vi "CALC_Fwd_adjust_TTL_pulse_length_according_to_stim_type_2.vi"(9 "Condition":refnum<class "Reward_Condition.lvclass">, 10 "Calibration parameters":T1 {"True frame time, s" format="%.10g"; "Disp. calibration info"."Speed, µl per ms" format="%.3g"; "True FPS" format="%.10g"; "Timing calibration sw/hw" format="%.10g"}, 11 "TTL pulse length ref in":refnum<vi>) -> ()   [LabVIEW 2018, in "Tracker.lvlib"]
uses:
  Tracker.lvlib
  Controls/CTL_Calibration_parameters.ctl
  Controls/CTL_Dispenser_calibration_info.ctl
  Classes/Reward_Condition/Reward_Condition.lvclass
  Classes/Reward_Condition/Reward_Condition.lvclass/Reward_Condition.ctl
  Classes/Reward_Condition/Read Response destination.vi
  Classes/Reward_Condition/Read Response length, ms.vi
  Classes/Reward_Condition/Read Response type.vi
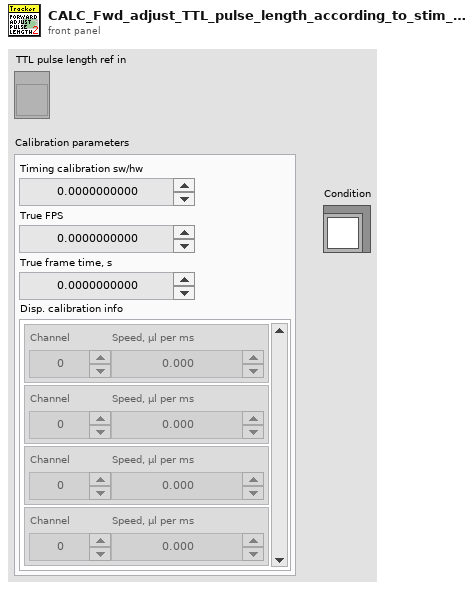
[diagram p1: front panel]
types:
  T1 = typedef "Tracker.lvlib/CTL_Calibration_parameters.ctl" = cluster{"Timing calibration sw/hw":dbl, "True FPS":dbl, "True frame time, s":dbl, "Disp. calibration info":T2}
  T2 = typedef "Tracker.lvlib/CTL_Dispenser_calibration_info.ctl" = cluster{"Channel":u8, "Speed, µl per ms":dbl}[]
  T3 = enum16{"None", "Port 1", "Port 2", "Port 3", "Port 4"}
  T4 = enum16{"None", "Air puff", "Liquid reward", "TTL pulse", "TTL trigger"}
  T5 = enum8{"Enabled", "Disabled", "Disabled and Grayed Out"}
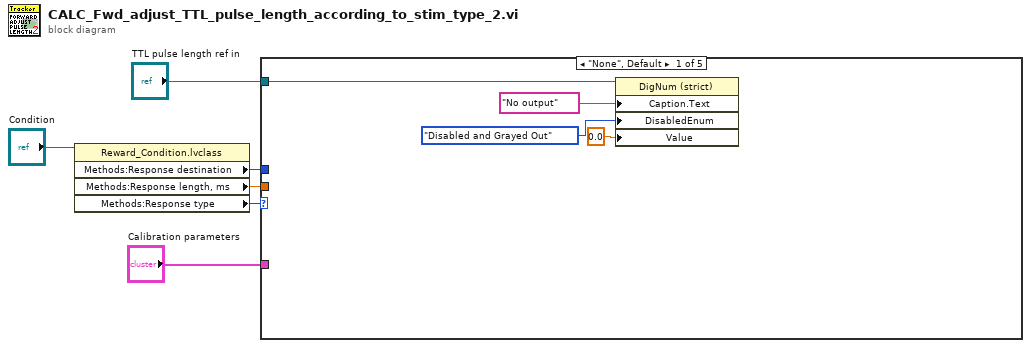
[diagram p0: block diagram]
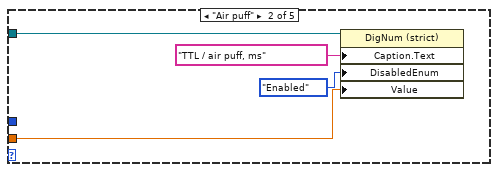
[diagram p2: hidden frame]
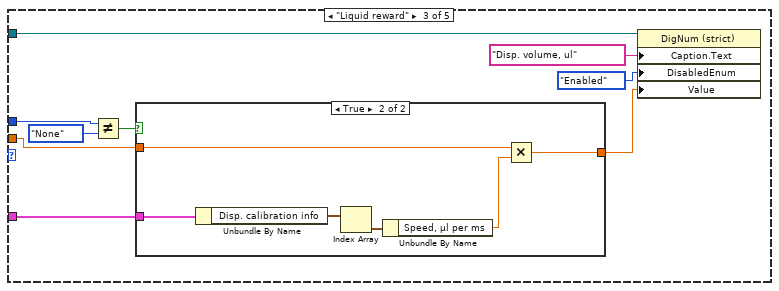
[diagram p3: hidden frame]
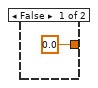
[diagram p4: hidden frame]
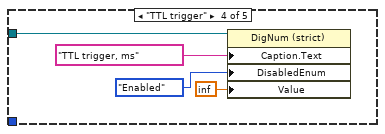
[diagram p5: hidden frame]
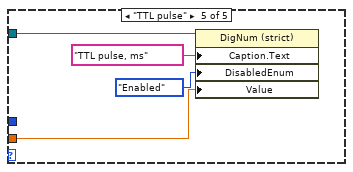
[diagram p6: hidden frame]
diagram:
  n1 = property class="Reward_Condition.lvclass"(reference="Condition") -> ("Methods:Response destination"=w2:T3, "Methods:Response length, ms"=w3:dbl, "Methods:Response type"=w1:T4)  [unwired: 1 in, 2 out]
  n2 = case shown="\"None\", Default" w1 {
    tunnel: w3 -> [_ w11 w22 _ w35]
    tunnel: "Calibration parameters" -> [_ _ w23 _ _]
    tunnel: w2 -> [_ _ w18 _ _]
    tunnel: "TTL pulse length ref in" -> [w8 w12 w19 w32 w36]
    frame "None", Default {
      n3 = property on="Property Node" class="DigNum (strict)"(reference=w8, "Caption.Text"="No output", "DisabledEnum"=T5."Disabled and Grayed Out" ("Disabled"), "Value"=0.0 ("TTL pulse length, ms")) -> ()  [unwired: 1 in, 2 out]
    }
    frame "Air puff" {
      n4 = property on="Property Node" class="DigNum (strict)"(reference=w12, "Caption.Text"="TTL / air puff, ms", "DisabledEnum"=T5."Enabled" ("Disabled"), "Value"=w11) -> ()  [unwired: 1 in, 2 out]
    }
    frame "Liquid reward" {
      n5 = Not Equal?(x=w18, y=T3."None") -> (x != y?=w16:bool)
      n6 = case shown="True" w16 {
        tunnel: w23 -> [_ w30]
        tunnel: w22 -> [_ w26]
        tunnel: [0.0 w25] -> w15
        frame False {
        }
        frame True {
          n7 = Unbundle By Name(w30) -> ("Disp. calibration info"=w29:T2)
          n8 = Index Array(array=w29) -> (element=w28:cluster{"Channel":u8, "Speed, µl per ms":dbl})  [unwired: 1 in]
          n9 = Unbundle By Name(w28) -> ("Speed, µl per ms"=w27:dbl)
          n10 = Multiply(x=w26, y=w27) -> (x*y=w25:dbl)
        }
      }
      n11 = property on="Property Node" class="DigNum (strict)"(reference=w19, "Caption.Text"="Disp. volume, ul", "DisabledEnum"=T5."Enabled" ("Disabled"), "Value"=w15) -> ()  [unwired: 1 in, 2 out]
    }
    frame "TTL trigger" {
      n12 = property on="Property Node" class="DigNum (strict)"(reference=w32, "Caption.Text"="TTL trigger, ms", "DisabledEnum"=T5."Enabled" ("Disabled"), "Value"=inf) -> ()  [unwired: 1 in, 2 out]
    }
    frame "TTL pulse" {
      n13 = property on="Property Node" class="DigNum (strict)"(reference=w36, "Caption.Text"="TTL pulse, ms", "DisabledEnum"=T5."Enabled" ("Disabled"), "Value"=w35) -> ()  [unwired: 1 in, 2 out]
    }
  }
